vi "Current K6221 Coarse.vi"() -> ()   [LabVIEW 2021]
panel:
  out "K6221 Coarse Current":dbl
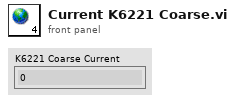
[diagram p1: front panel]
diagram:
